vi "2_Waveform_Signal_Regression_Multi_Output(Inference).vi"() -> ()   [LabVIEW 2020]
uses:
  <vilib>/Ngene/DeepLTK/Toolkit/NN_Network/Controls/NN_Save_Before_Destroy_Options.ctl
  <vilib>/Ngene/DeepLTK/Toolkit/NN_Layers/Layers/Input/API/NN_Layer_Set_Out(Input1D_idx).vi
  <vilib>/Ngene/DeepLTK/Toolkit/Deep_Learning_Toolkit_by_Ngene.lvlib
  <vilib>/measure/NI_MABase.lvlib
panel:
  out "Phase":cluster{"Original Value":dbl, "Frequency":dbl}(graph)={"Original Value"=217.09099978208542, "Frequency"=208.85496183206106}
  out "Amplitude":cluster{"Original Value":dbl, "Frequency":dbl}(graph)={"Original Value"=8.13217664361, "Frequency"=7.128244274809161}
  in  "Noise":dbl(slide) scale=0.0..5.0
  in  "Offset":dbl(slide)=0.534351145038169 scale=-10.0..10.0
  in  "Phase":dbl(slide)=208.85496183206106 scale=0.0..360.0
  in  "Amplitude":dbl(slide)=7.128244274809161 scale=0.1..10.0
  in  "Frequency":dbl(slide)=73.20610687022901 scale=10.0..100.0
  out "Offset":cluster{"Original Value":dbl, "Frequency":dbl}(graph)={"Original Value"=0.6723126769065857, "Frequency"=0.534351145038169}
  out "Phase\n(Predicted)":dbl=217.09099978208542 format="%#_3g"
  out "Ampitude\n(Predicted)":dbl=8.13217664361 format="%#_3g"
  out "Frequency\n(Predicted)":dbl=74.96004462242126 format="%#_3g"
  out "Frequency":cluster{"Original Value":dbl, "Frequency":dbl}(graph)={"Original Value"=74.96004462242126, "Frequency"=73.20610687022901}
  out "Offset\n(Predicted)":dbl=0.6723126769065857 format="%#_3g"
  out "Generated WaveForm":waveform(dbl)(graph)={"t0"=timestamp(0 s since 1904-01-01), "dt"=0.001, "Y"=[-6.593893129770992, -6.593893129770992, -6.593893129770992, -6.593893129770992, -6.593893129770992, -6.593893129770992, 7.66259541984733, 7.66259541984733, 7.66259541984733, 7.66259541984733, 7.66259541984733, 7.66259541984733, -6.593893129770992, -6.593893129770992, -6.593893129770992, -6.593893129770992, -6.593893129770992, -6.593893129770992, -6.593893129770992, -6.593893129770992, 7.66259541984733, 7.66259541984733, 7.66259541984733, 7.66259541984733, 7.66259541984733, 7.66259541984733, -6.593893129770992, -6.593893129770992, -6.593893129770992, -6.593893129770992, -6.593893129770992, -6.593893129770992, -6.593893129770992, -6.593893129770992, 7.66259541984733, 7.66259541984733, 7.66259541984733, 7.66259541984733, 7.66259541984733, 7.66259541984733, -6.593893129770992, -6.593893129770992, -6.593893129770992, -6.593893129770992, -6.593893129770992, -6.593893129770992, -6.593893129770992, 7.66259541984733, 7.66259541984733, 7.66259541984733, 7.66259541984733, 7.66259541984733, 7.66259541984733, -6.593893129770992, -6.593893129770992, -6.593893129770992, -6.593893129770992, -6.593893129770992, -6.593893129770992, -6.593893129770992, -6.593893129770992, 7.66259541984733, 7.66259541984733, 7.66259541984733, 7.66259541984733, 7.66259541984733, 7.66259541984733, -6.593893129770992, -6.593893129770992, -6.593893129770992, -6.593893129770992, -6.593893129770992, -6.593893129770992, -6.593893129770992, -6.593893129770992, 7.66259541984733, 7.66259541984733, 7.66259541984733, 7.66259541984733, 7.66259541984733, 7.66259541984733, -6.593893129770992, -6.593893129770992, -6.593893129770992, -6.593893129770992, -6.593893129770992, -6.593893129770992, -6.593893129770992, 7.66259541984733, 7.66259541984733, 7.66259541984733, 7.66259541984733, 7.66259541984733, 7.66259541984733, -6.593893129770992, -6.593893129770992, -6.593893129770992, -6.593893129770992, -6.593893129770992, -6.593893129770992]}
  in  "Signal Type":T1(ring)=enum."Square Wave"
  in  "Weight File Path":path=path "D:/Ngene/GitHub/deepltk_examples/2_Waveform_Processing/23_Waveform_Signal_Regression_Multi_Output/working/WF_Regression_Multi_Output/WF_Regression_Multi_Output_weights_23_10_18__18_42_11.bin"
  in  "Network Configuration File Path":path=path "D:/Ngene/GitHub/deepltk_examples/2_Waveform_Processing/23_Waveform_Signal_Regression_Multi_Output/working/WF_Regression_Multi_Output/WF_Regression_Multi_Output_net_cfg_23_10_18__18_42_11.cfg"
  in  "Stop":bool
  # "Overview: Demonstrates the usage of DeepLTK for loading the model pretrained for multioutput waveform signal regression and running for inference.\nRequirements: DeepLTK - Deep Learning Toolkit for LabVIEW (https://www.ngene.co/deep-learning-toolkit-for-labview)\nInstructions:\n1. Provide Network Configuration File Path and Weight File Path generated from training example.\n2. Run the VI\n3. Input Waveform parameters and observe the predicted frequency against reference value.\n4. Press the Stop button to stop the VI.\n\nMore Examples:  https://github.com/ngenehub/deepltk_examples"
  # "Waveform Signal Regression (Inference)\nMultiple Property Prediction"
  # "Predicted Properties vs Reference"
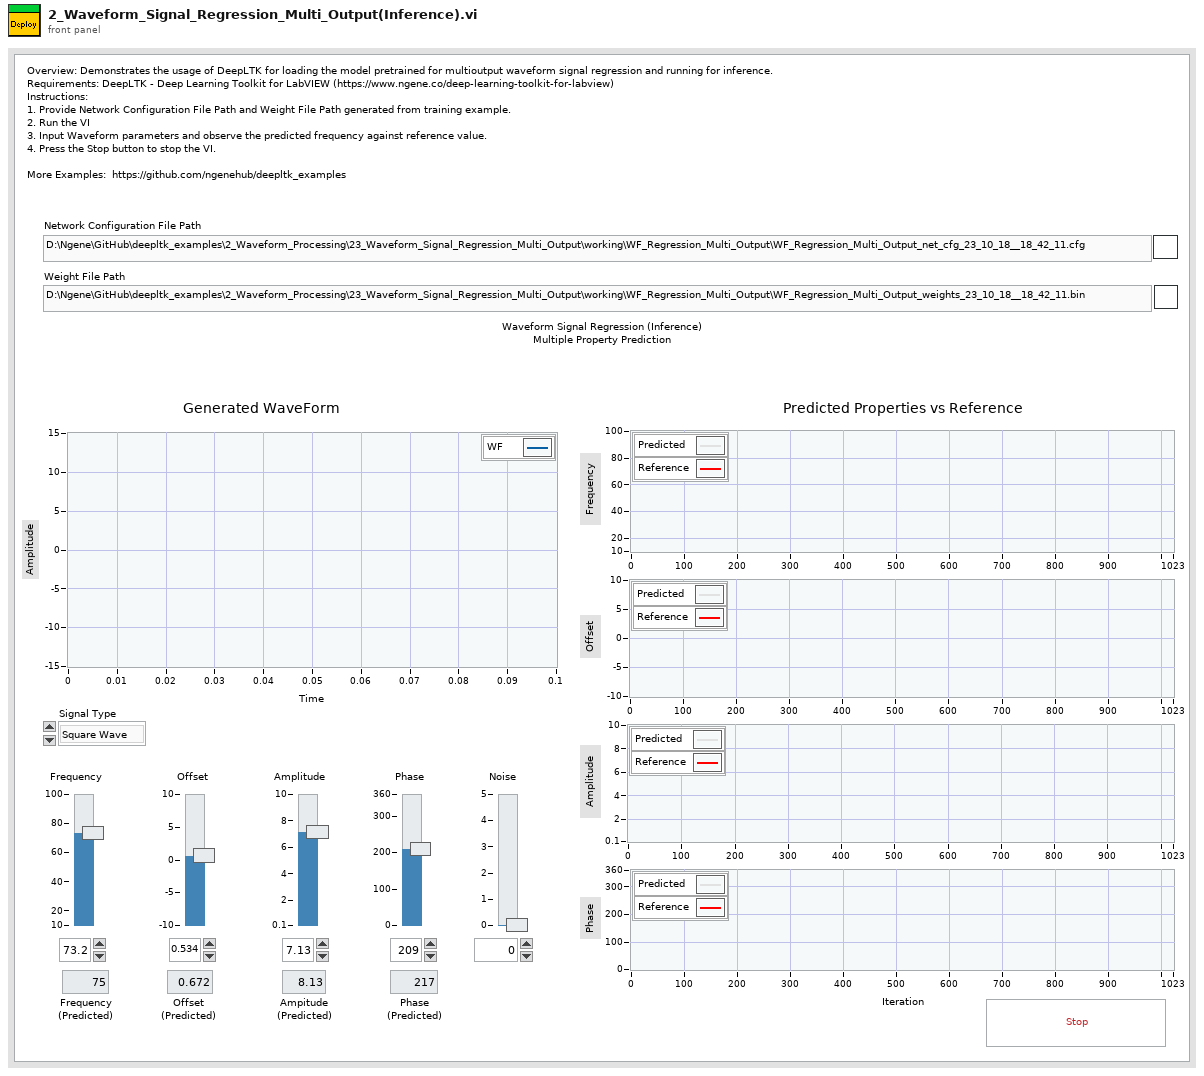
[diagram p1: front panel]
types:
  T1 = enum16{"Sine Wave", "Triangle Wave", "Square Wave", "Sawtooth Wave"}
  T2 = typedef "Deep_Learning_Toolkit_by_Ngene.lvlib/NN_Save_Before_Destroy_Options.ctl" = cluster{"CFG?":bool, "Weights?":bool, "Render?":bool}
  T3 = typedef "Deep_Learning_Toolkit_by_Ngene.lvlib/NN_Config_Params.ctl" = cluster{"Name":string, "mBatch":i32, "NN_Train_Params":T4, "LR_Decay_Policy":T7, "Labels":string[], "Loss":T9}
  T4 = typedef "Deep_Learning_Toolkit_by_Ngene.lvlib/NN_Train_Params.ctl" = cluster{"Optimizer":T5, "Beta_1":sgl, "Beta_2":sgl, "Weight Decay(L1)":sgl, "Weight Decay(L2)":sgl, "Data_Sampling":T6}
  T5 = typedef "Deep_Learning_Toolkit_by_Ngene.lvlib/NN_Train_Optimizer.ctl" = enum16{"SGD", "Adam", "Adagrad", "Adadelta", "RMSProp", "Nesterov"}
  T6 = typedef "Deep_Learning_Toolkit_by_Ngene.lvlib/NN_Train_Data_Sampling.ctl" = enum16{"Random", "Sequential"}
  T7 = typedef "Deep_Learning_Toolkit_by_Ngene.lvlib/NN_LR_Policy_Cfg.ctl" = cluster{"Policy_Type":T8, "LR0":dbl, "k":sgl, "WarmUp_Policy":enum16{"Step", "Ramp"}, "WarmUp_Iter":i32, "WarmUp_Ratio":sgl}
  T8 = typedef "Deep_Learning_Toolkit_by_Ngene.lvlib/NN_LR_Policy_Type.ctl" = enum16{"Manual", "Step", "Exp", "1/t"}
  T9 = typedef "Deep_Learning_Toolkit_by_Ngene.lvlib/NN_Loss_Config_Params.ctl" = cluster{"Loss_Type":T10, "Loss_Conf_Params":variant}
  T10 = typedef "Deep_Learning_Toolkit_by_Ngene.lvlib/NN_Loss_Type.ctl" = enum16{"None", "MSE", "CrossEntropy", "YOLO_v2"}
  T11 = typedef "Deep_Learning_Toolkit_by_Ngene.lvlib/NN_Layer_Config_Params.ctl" = cluster{"Layer_Type":T12, "Layer_Conf_Params":variant}
  T12 = typedef "Deep_Learning_Toolkit_by_Ngene.lvlib/NN_Layer_Type.ctl" = enum16{"Input1D", "Input3D", "Conv2D", "Conv2D_Adv", "MaxPool", "AvgPool", "UpSample", "DropOut3D", "ShortCut", "Concat", "SoftMax3D", "FC", "DropOut", "Softmax", "Flatten", "YOLO_v2", "Unsupported"}
  T13 = typedef "Deep_Learning_Toolkit_by_Ngene.lvlib/NN.ctl" = cluster{"Name":string, "No of Layers":i32, "mBatch":i32, "Layers":T14[], "Dimty":T15, "Dims_In":T16, "Dims_Out":T16, "Working_Dir":path, "Train?":bool, "Train_Params":T4, "LR_Update_Policy":T7, "Session Data":T17, "Ground_truth":T18, "NNg_hdls":T20, "NN_Device":T21, "GPU Id":i32, "Labels":string[], "Receptive Field":T22[], "Loss_Type":T10, "Loss_Cfg_Prms":variant}
  T14 = typedef "Deep_Learning_Toolkit_by_Ngene.lvlib/NN_Layer_ref.ctl" = refnum<data-value>
  T15 = typedef "Deep_Learning_Toolkit_by_Ngene.lvlib/NN_In_Out_Dim-ty.ctl" = enum8{"In1D_Out1D", "In3D_Out1D", "In3D_Out3D", "In3D_OutBBox"}
  T16 = typedef "Deep_Learning_Toolkit_by_Ngene.lvlib/NN_Dims(C,H,W).ctl" = cluster{"C":i32, "H":i32, "W":i32}
  T17 = typedef "Deep_Learning_Toolkit_by_Ngene.lvlib/NN_Train_Session_Data.ctl" = cluster{"Epochs":sgl, "Tot_Iter":i32, "LR":sgl, "LR_iter":i32}
  T18 = typedef "Deep_Learning_Toolkit_by_Ngene.lvlib/NN_Ground_truth.ctl" = cluster{"Y":variant, "Y_idx":T19}
  T19 = typedef "Deep_Learning_Toolkit_by_Ngene.lvlib/NN_Data_ref(1D_I32).ctl" = refnum<data-value>
  T20 = typedef "Deep_Learning_Toolkit_by_Ngene.lvlib/nng_cuda_handles.ctl" = cluster{"cudnn":u64, "cublas":u64, "stream":u64, "curand":u64}
  T21 = typedef "Deep_Learning_Toolkit_by_Ngene.lvlib/NN_Device.ctl" = enum16{"CPU", "GPU"}
  T22 = typedef "Deep_Learning_Toolkit_by_Ngene.lvlib/NN_Dims(V,H).ctl" = cluster{"V":i32, "H":i32}
  T23 = typedef "Deep_Learning_Toolkit_by_Ngene.lvlib/NN_Layer.ctl" = cluster{"Name":string, "Layer_Data":variant, "Layer_Type":T12, "Dims_In":T16, "Layers_In":variant, "Dims_Out":T16, "Layers_Out":variant, "Metrics":T24, "GPU_Data":variant, "mBatch":i32, "NN_Device":T21, "NNg_hdls":T20, "Train?":bool, "Dimty":T25, "RecptField":T26}
  T24 = typedef "Deep_Learning_Toolkit_by_Ngene.lvlib/NN_Layer_Metrics.ctl" = cluster{"Data":dbl, "Params":dbl, "Ops":dbl}
  T25 = typedef "Deep_Learning_Toolkit_by_Ngene.lvlib/NN_Layer_Dimty.ctl" = enum16{"1D", "3D"}
  T26 = typedef "Deep_Learning_Toolkit_by_Ngene.lvlib/NN_Layer_RF_State.ctl" = cluster{"Dims":T22, "J":T22}
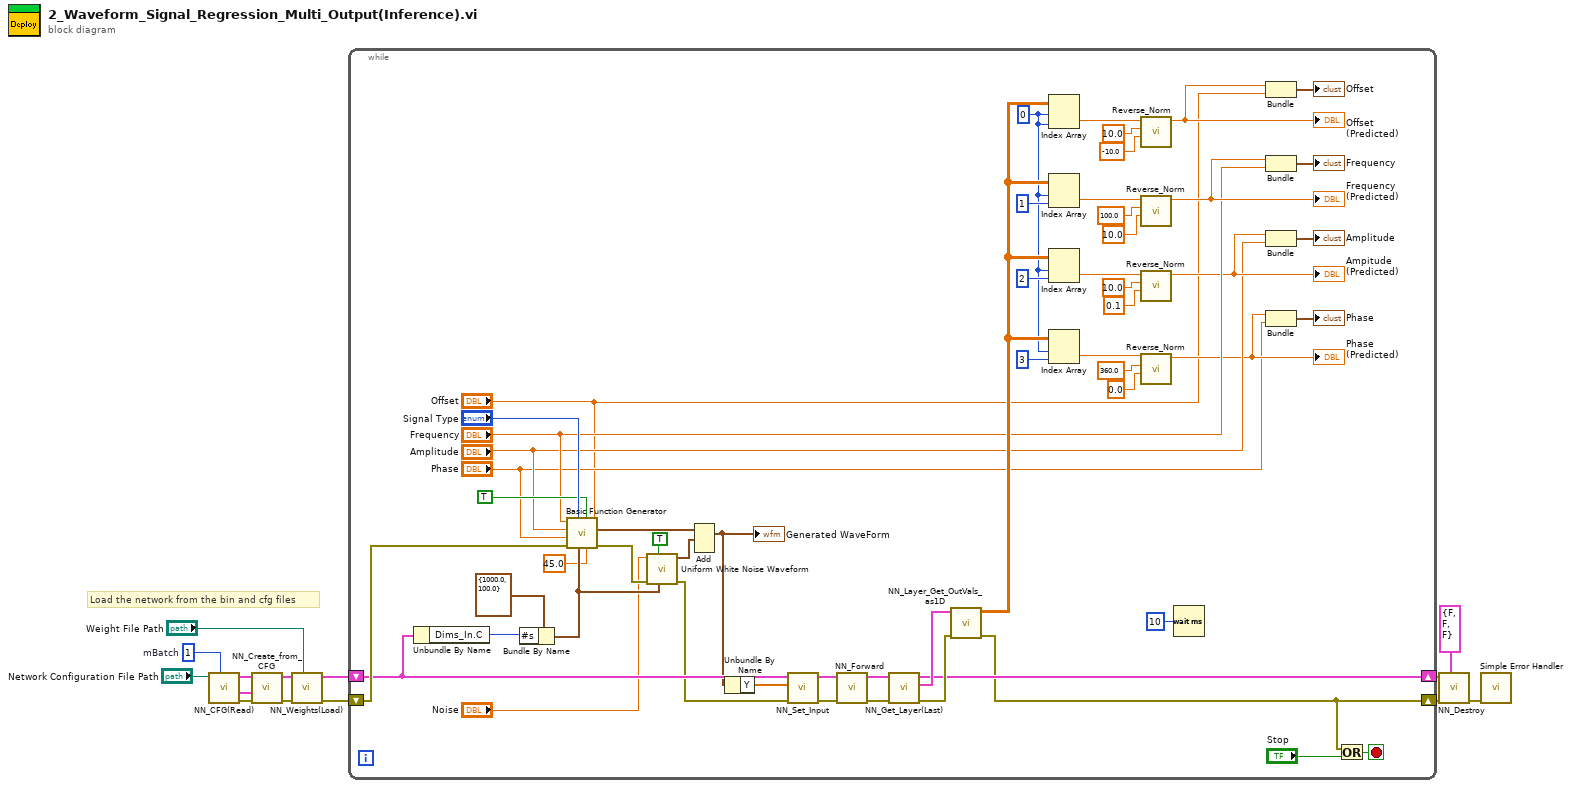
[diagram p0: block diagram]
diagram:
  w2 = 1  # mBatch
  # "Load the network from the bin and cfg files"
  n1 = call <vilib>:"NN_CFG(Read).vi"("mBatch"=w2, "CFG file path"="Network Configuration File Path") -> ("error out"=w8:errorcluster, "Net_Cfg"=w9:T3, "Layer_Cfg"=w7:T11[])  [unwired: 7 in]
  n2 = call <vilib>:"NN_Create_from_CFG.vi"("error in (no error)"=w8, "Net_Cfg"=w9, "Layer_Cfg"=w7) -> ("error out"=w11:errorcluster, "NN out"=w6:T13)  [unwired: 7 in]
  n3 = call <vilib>:"NN_Weights(Load).vi"("Weight File Path"="Weight File Path", "error in (no error)"=w11, "NN in"=w6) -> ("error out"=w5:errorcluster, "NN out"=w4:T13)  [unwired: 7 in]
  n4 = while {
    shift-right: [w16] -> w14
    shift-left: w5 -> [w70]
    shift-right: [w57] -> w13
    shift-left: w4 -> [w59]
    stop <- w17 stop-if-true
    w31 = 0 ("index (row)")
    n5 = Unbundle By Name(w59) -> ("Dims_In.C"=w58:i32)
    n6 = Bundle By Name(cluster=cluster{"Fs":dbl, "#s":dbl} {"Fs"=1000.0, "#s"=100.0} ("sampling info"), "#s"=w58) -> (w52:cluster{"Fs":dbl, "#s":dbl})
    n7 = call <vilib>:"Basic Function Generator.vi"("offset"="Offset", "square wave duty cycle (%)"=45.0, "reset signal"=TRUE, "sampling info"=w52, "signal type"="Signal Type", "error in (no error)"=w70, "phase"="Phase", "amplitude"="Amplitude", "frequency"="Frequency") -> ("error out"=w53:errorcluster, "signal out"=w55:waveform(dbl))  [unwired: 1 out]
    n8 = call <vilib>:"Uniform White Noise Waveform.vi"("sampling info"=w52, "reset signal"=TRUE, "error in (no error)"=w53, "amplitude"="Noise") -> ("error out"=w15:errorcluster, "signal out"=w50:waveform(dbl))  [unwired: 6 in]
    n9 = Add(1:w50, 2:w55) -> (0:w51:waveform(dbl))  [unwired: 1 in, 1 out]
    "Generated WaveForm" <- w51
    n10 = Unbundle By Name(w51) -> ("Y"=w63:dbl[])
    n11 = call-poly <vilib>:"NN_Set_Input.vi"("error in (no error)"=w15, "Data_In(1D_SGL)"=w63, "NN In"=w59) -> ("error out"=w69:errorcluster, "NN Out"=w66:T13)  [unwired: 7 in]
    n12 = call <vilib>:"NN_Forward.vi"("error in (no error)"=w69, "NN in"=w66) -> ("error out"=w68:errorcluster, "NN out"=w67:T13)  [unwired: 6 in, 2 out]
    n13 = call <vilib>:"NN_Get_Layer(Last).vi"("error in (no error)"=w68, "NN in"=w67) -> ("error out"=w65:errorcluster, "Last_Layer"=w64:T23, "NN out"=w57:T13)  [unwired: 6 in, 1 out]
    n14 = call <vilib>:"NN_Layer_Get_OutVals_as1D.vi"("error in (no error)"=w65, "Layer"=w64) -> ("error out"=w16:errorcluster, "Out(as1D)"=w44:sgl[][])  [unwired: 8 in]
    n15 = Index Array(array=w44, index (row)=w31, index (col)=w31) -> (element=w43:sgl)
    n16 = Index Array(array=w44, index (row)=w31, index (col)=1 ("index (row)")) -> (element=w40:sgl)
    n17 = Index Array(array=w44, index (row)=w31, index (col)=2 ("index (row)")) -> (element=w37:sgl)
    n18 = Index Array(array=w44, index (row)=w31, index (col)=3 ("index (row)")) -> (element=w34:sgl)
    n19 = call "Reverse_Norm.vi"("Min"=-10.0, "Max"=10.0, "Norm Value"=w43) -> ("Original Value"=w27:dbl)  [unwired: 8 in]
    "Offset\n(Predicted)" <- w27
    n20 = call "Reverse_Norm.vi"("Min"=10.0, "Max"=100.0, "Norm Value"=w40) -> ("Original Value"=w29:dbl)  [unwired: 8 in]
    "Frequency\n(Predicted)" <- w29
    n21 = call "Reverse_Norm.vi"("Min"=0.1, "Max"=10.0, "Norm Value"=w37) -> ("Original Value"=w23:dbl)  [unwired: 8 in]
    "Ampitude\n(Predicted)" <- w23
    n22 = call "Reverse_Norm.vi"("Min"=0.0, "Max"=360.0, "Norm Value"=w34) -> ("Original Value"=w20:dbl)  [unwired: 8 in]
    "Phase\n(Predicted)" <- w20
    n23 = Wait (ms)(milliseconds to wait=u32 10) -> ()  [unwired: 1 out]
    n24 = Bundle("Original Value"=w27, "Offset"="Offset") -> (→"Offset":cluster{"Original Value":dbl, "Offset":dbl})  [unwired: 1 in]
    n25 = Bundle("Original Value"=w29, "Frequency"="Frequency") -> (→"Frequency":cluster{"Original Value":dbl, "Frequency":dbl})  [unwired: 1 in]
    n26 = Bundle("Original Value"=w23, "Amplitude"="Amplitude") -> (→"Amplitude":cluster{"Original Value":dbl, "Amplitude":dbl})  [unwired: 1 in]
    n27 = Bundle("Original Value"=w20, "Phase"="Phase") -> (→"Phase":cluster{"Original Value":dbl, "Phase":dbl})  [unwired: 1 in]
    n28 = Or(x=w16, y="Stop") -> (x .or. y?=w17:bool)
  }
  n29 = call <vilib>:"NN_Destroy.vi"("Save (T, T, T)"=T2 {"CFG?"=FALSE, "Weights?"=FALSE, "Render?"=FALSE}, "error in (no error)"=w14, "NN in"=w13) -> ("error out"=w1:errorcluster)  [unwired: 8 in]
  n30 = call <vilib>:"Simple Error Handler.vi"("error in (no error)"=w1) -> ()  [unwired: 4 in, 5 out]
